vi "FS Sketch Text.vi"(8 "Sketch/Body #":i32=1, 9 "text":T2={"left"=0.0, "top"=2.0, "right"=2.0, "bottom"=0.0, "String"="Text"}, 10 "Sketch Plane":T1, 11 "Feature In":string="FeatureScript 1247;\nimport(path : \"onshape/std/geometry.fs\", version : \"1247.0\");\n\nannotation { \"Feature Type Name\" : \"LabVIEW Feature\" }\nexport const myFeature = defineFeature(function(context is Context, id is Id, definition is map)\n    precondition\n    {\n        // Define the parameters of the feature type\n    }\n    {\n               fEllipsoid(context, id + \"ellipsoid1\", {\n                \"center\" : vector(-0, -7, 8) * inch,\n                \"radius\" : vector(3, 3, 3) * inch,\n        });\n        var sketch1 = newSketch(context, id + \"sketch1\", {\n                \"sketchPlane\" : qCreatedBy(makeId(\"Top\"), EntityType.FACE)\n        });\n        // Create sketch entities here\n        skText(sketch1, \"text1\", {\n                \"text\" : \"N\",\n                \"fontName\" : \"OpenSans-Regular.ttf\",\n                \"firstCorner\" : vector(-0.500000, 4.000000) * inch,\n                \"secondCorner\" : vector(0.500000, 3.000000) * inch\n        });\n        skSolve(sketch1);\n        var sketch2 = newSketch(context, id + \"sketch2\", {\n                \"sketchPlane\" : qCreatedBy(makeId(\"Top\"), EntityType.FACE)\n        });\n        // Create sketch entities here\n        skText(sketch2, \"text1\", {\n                \"text\" : \"S\",\n                \"fontName\" : \"OpenSans-Regular.ttf\",\n                \"firstCorner\" : vector(-0.500000, -4.000000) * inch,\n                \"secondCorner\" : vector(0.500000, -3.000000) * inch\n        });\n        skSolve(sketch2);\n        var sketch3 = newSketch(context, id + \"sketch3\", {\n                \"sketchPlane\" : qCreatedBy(makeId(\"Top\"), EntityType.FACE)\n        });\n        // Create sketch entities here\n        skText(sketch3, \"text1\", {\n                \"text\" : \"E\",\n                \"fontName\" : \"OpenSans-Regular.ttf\",\n                \"firstCorner\" : vector(3.000000, 0.500000) * inch,\n                \"secondCorner\" : vector(4.000000, -0.500000) * inch\n        });\n        skSolve(sketch3);\n// Define the function's action\n    });") -> (3 "Feature Out":string="FeatureScript 1247;\nimport(path : \"onshape/std/geometry.fs\", version : \"1247.0\");\n\nannotation { \"Feature Type Name\" : \"LabVIEW Feature\" }\nexport const myFeature = defineFeature(function(context is Context, id is Id, definition is map)\n    precondition\n    {\n        // Define the parameters of the feature type\n    }\n    {\n               fEllipsoid(context, id + \"ellipsoid1\", {\n                \"center\" : vector(-0, -7, 8) * inch,\n                \"radius\" : vector(3, 3, 3) * inch,\n        });\n        var sketch1 = newSketch(context, id + \"sketch1\", {\n                \"sketchPlane\" : qCreatedBy(makeId(\"Top\"), EntityType.FACE)\n        });\n        // Create sketch entities here\n        skText(sketch1, \"text1\", {\n                \"text\" : \"N\",\n                \"fontName\" : \"OpenSans-Regular.ttf\",\n                \"firstCorner\" : vector(-0.500000, 4.000000) * inch,\n                \"secondCorner\" : vector(0.500000, 3.000000) * inch\n        });\n        skSolve(sketch1);\n        var sketch2 = newSketch(context, id + \"sketch2\", {\n                \"sketchPlane\" : qCreatedBy(makeId(\"Top\"), EntityType.FACE)\n        });\n        // Create sketch entities here\n        skText(sketch2, \"text1\", {\n                \"text\" : \"S\",\n                \"fontName\" : \"OpenSans-Regular.ttf\",\n                \"firstCorner\" : vector(-0.500000, -4.000000) * inch,\n                \"secondCorner\" : vector(0.500000, -3.000000) * inch\n        });\n        skSolve(sketch2);\n        var sketch3 = newSketch(context, id + \"sketch3\", {\n                \"sketchPlane\" : qCreatedBy(makeId(\"Top\"), EntityType.FACE)\n        });\n        // Create sketch entities here\n        skText(sketch3, \"text1\", {\n                \"text\" : \"E\",\n                \"fontName\" : \"OpenSans-Regular.ttf\",\n                \"firstCorner\" : vector(3.000000, 0.500000) * inch,\n                \"secondCorner\" : vector(4.000000, -0.500000) * inch\n        });\n        skSolve(sketch3);\n        var sketch4 = newSketch(context, id + \"sketch4\", {\n                \"sketchPlane\" : qCreatedBy(makeId(\"Top\"), EntityType.FACE)\n        });\n        // Create sketch entities here\n        skText(sketch4, \"text1\", {\n                \"text\" : \"W\",\n                \"fontName\" : \"OpenSans-Regular.ttf\",\n                \"firstCorner\" : vector(-3.000000, 0.500000) * inch,\n                \"secondCorner\" : vector(-4.000000, -0.500000) * inch\n        });\n        skSolve(sketch4);\n// Define the function's action\n    });")   [LabVIEW 2019]
uses:
  <userlib>/Onshape Feature Funcrions/_SubVI/Sketch Plane.ctl
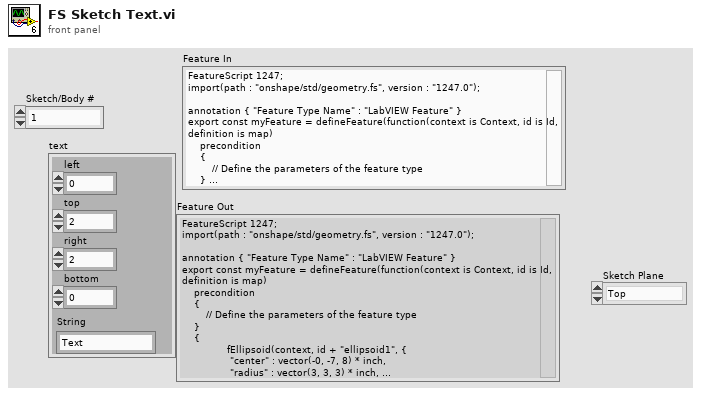
[diagram p1: front panel]
types:
  T1 = typedef "Sketch Plane.ctl" = enum16{"Top", "Front", "Right", "plane1", "plane2", "plane3"}
  T2 = cluster{"left":dbl, "top":dbl, "right":dbl, "bottom":dbl, "String":string}
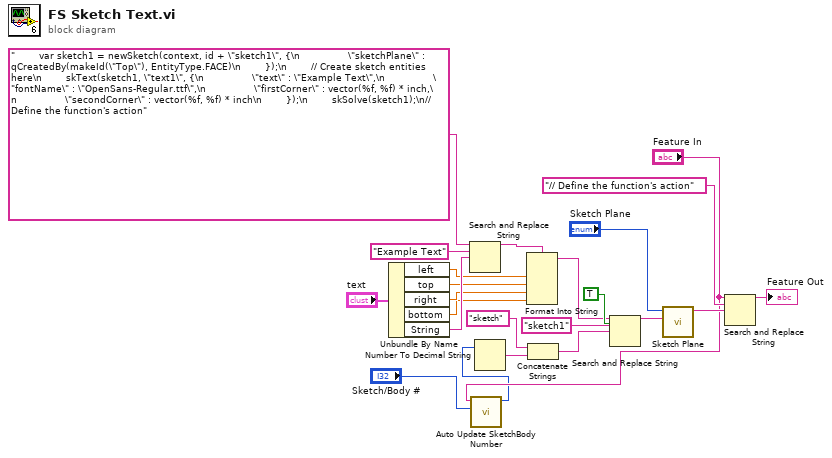
[diagram p0: block diagram]
diagram:
  n1 = Unbundle By Name("text") -> ("left"=w12:dbl, "top"=w11:dbl, "right"=w10:dbl, "bottom"=w9:dbl, "String"=w18:string)
  n2 = Search and Replace String(input string="        var sketch1 = newSketch(context, id + \"sketch1\", {\n                \"sketchPlane\" : qCreatedBy(makeId(\"Top\"), EntityType.FACE)\n        });\n        // Create sketch entities here\n        skText(sketch1, \"text1\", {\n                \"text\" : \"Example Text\",\n                \"fontName\" : \"OpenSans-Regular.ttf\",\n                \"firstCorner\" : vector(%f, %f) * inch,\n                \"secondCorner\" : vector(%f, %f) * inch\n        });\n        skSolve(sketch1);\n// Define the function's action" ("search string"), search string="Example Text" ("regular expression"), replace string=w18) -> (result string=w4:string)  [unwired: 5 in, 3 out]
  n3 = call "Auto Update SketchBody Number.vi"("Sketch # in"="Sketch/Body #", "Feature In"="Feature In") -> ("Sketch # out"=w1:i32)  [unwired: 8 in, 1 out]
  n4 = Number To Decimal String(number=w1) -> (decimal integer string=w13:string)  [unwired: 1 in]
  n5 = Format Into String(format string=w4, w12, w11, w10, w9) -> (resulting string=w8:string)  [unwired: 2 in, 1 out]
  n6 = Concatenate Strings("sketch" ("regular expression"), w13) -> (w17:string)
  n7 = Search and Replace String(replace all?=TRUE ("replace all? (F)"), input string=w8, search string="sketch1" ("regular expression"), replace string=w17) -> (result string=w7:string)  [unwired: 4 in, 3 out]
  n8 = call <userlib>:"Sketch Plane.vi"("result string in"=w7, "Sketch Plane"="Sketch Plane") -> ("result string out"=w5:string)  [unwired: 9 in]
  n9 = Search and Replace String(input string="Feature In", search string="// Define the function's action", replace string=w5) -> (result string=→"Feature Out":string)  [unwired: 5 in, 3 out]
